vi "Configure PRACH Settings.vi"(6 "Zero Correlation Zone (0)":i32, 7 "Logical Root Sequence (0)":i32, 8 "error in (no error)":errorcluster, 9 "Configuration Index (17)":i32=17, 10 "Instance (1)":T1=1, 11 "VISA resource name":refnum<visa-resource-name>) -> (0 "error out":errorcluster, 3 "VISA resource name out":refnum<visa-resource-name>)   [LabVIEW 2020, in "Rohde&Schwarz CMWXP NR FR1 Measurement.lvlib"]
doc: "The VI sets PRACH configuration index, Logical Root Sequence and Zero Correction Zone.\n\nAttributes:\nRSCMWXPNRFR1M_ATTR_PRACH_CONFIGURATION_INDEX\nRSCMWXPNRFR1M_ATTR_PRACH_LOGICAL_ROOT_SEQUENCE\nRSCMWXPNRFR1M_ATTR_PRACH_ZERO_CORRELATION_ZONE\n\nRemote-control commands:\nCONFigure:NRSub:MEAS<i>:PRACh:PCINdex\nCONFigure:NRSub:MEAS<i>:PRACh:LRSindex\nCONFigure:NRSub:MEAS<i>:PRACh:ZCZone"
uses:
  <instrlib>/Rohde&Schwarz CMWXP NR FR1 Measurement/Rohde&Schwarz CMWXP NR FR1 Measurement.lvlib
  <instrlib>/Rohde&Schwarz CMWXP NR FR1 Measurement/Private/_Instance.ctl
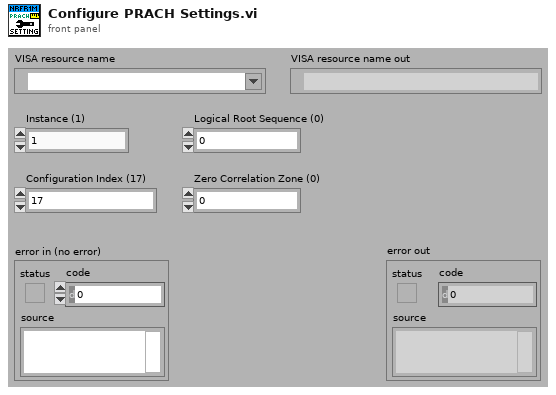
[diagram p1: front panel]
types:
  T1 = typedef "Rohde&Schwarz CMWXP NR FR1 Measurement.lvlib/_Instance.ctl" = i32
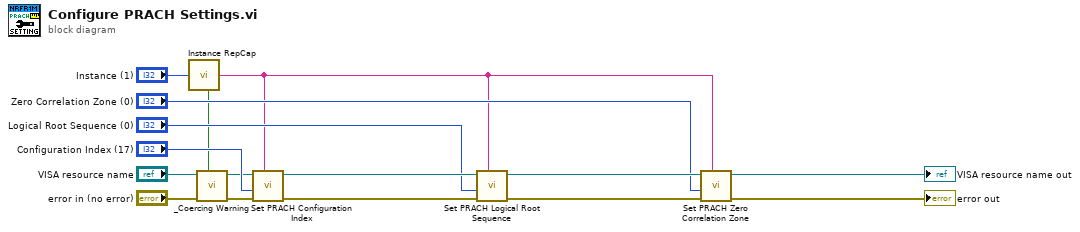
[diagram p0: block diagram]
diagram:
  n1 = call <instrlib>:"Instance RepCap.vi"("Instance In"="Instance (1)") -> ("In Range?"=w2:bool, "RepCap Identifier Out"=w1:string)  [unwired: 1 in]
  n2 = call <instrlib>:"_Coercing Warning.vi"("In Range?"=w2, "error in (no error)"="error in (no error)", "VISA resource name"="VISA resource name") -> ("error out"=w4:errorcluster, "VISA resource name out"=w3:refnum<visa-resource-name>)  [unwired: 7 in]
  n3 = call "Set PRACH Configuration Index"("Repeated Capabilities"=w1, "error in (no error)"=w4, "PRACH Configuration Index (0)"="Configuration Index (17)", "instrument handle"=w3) -> ("error out"=w14:errorcluster, "instrument handle out"=w15:refnum<visa-resource-name>)  [unwired: 6 in]
  n4 = call "Set PRACH Logical Root Sequence"("Repeated Capabilities"=w1, "error in (no error)"=w14, "PRACH Logical Root Sequence (0)"="Logical Root Sequence (0)", "instrument handle"=w15) -> ("error out"=w9:errorcluster, "instrument handle out"=w10:refnum<visa-resource-name>)  [unwired: 6 in]
  n5 = call "Set PRACH Zero Correlation Zone"("Repeated Capabilities"=w1, "error in (no error)"=w9, "PRACH Zero Correlation Zone (0)"="Zero Correlation Zone (0)", "instrument handle"=w10) -> ("error out"=→"error out":errorcluster, "instrument handle out"=→"VISA resource name out":refnum<visa-resource-name>)  [unwired: 6 in]
